vi "AI Read AFR.vi"(8 "Analog In":dbl[][](array[numeric]), 9 "Avg Point":i16[](array[numeric]), 10 "Intercept":dbl[](array[numeric]), 11 "Slope":dbl[](array[numeric])) -> (3 "Analog Out":T1)   [LabVIEW 2015]
uses:
  <vilib>/Analysis/baseanly.llb/Mean (DBL).vi
  <vilib>/Analysis/NI_AALBase.lvlib
  <vilib>/ptbypt/NI_PtbyPt.lvlib
panel:
  in  "Cluster":T1
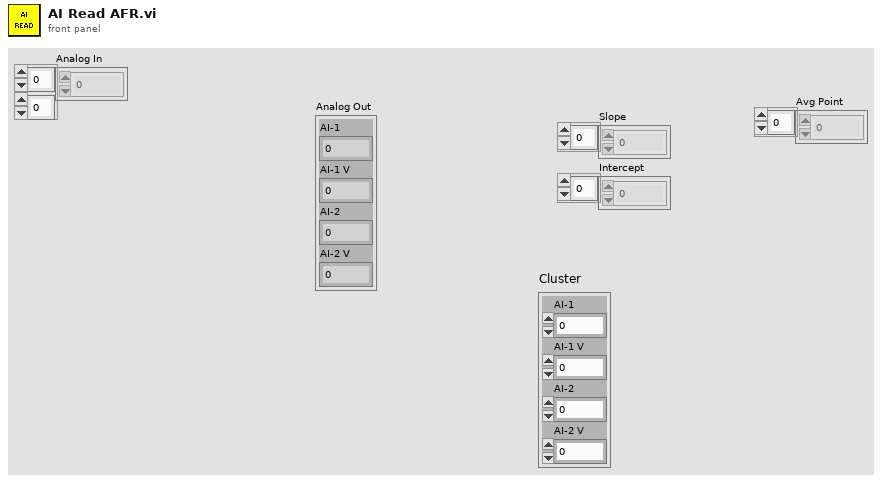
[diagram p1: front panel]
types:
  T1 = cluster{"AI-1":dbl, "AI-1 V":dbl, "AI-2":dbl, "AI-2 V":dbl}
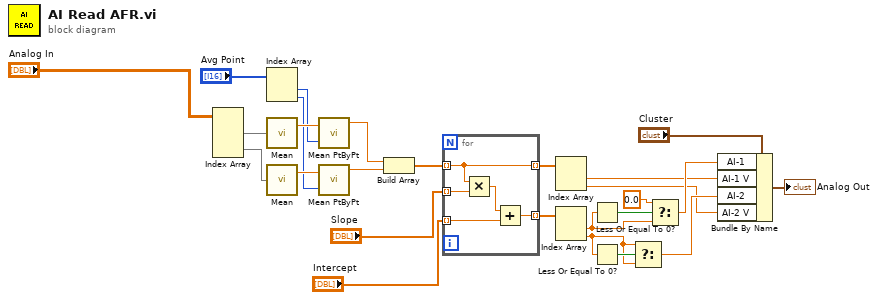
[diagram p0: block diagram]
diagram:
  n1 = Index Array(array="Analog In") -> (element #1=w4:dbl[], element #2=w3:dbl[])  [unwired: 4 in]
  n2 = Index Array(array="Avg Point") -> (element #1=w24:i16, element #2=w23:i16)  [unwired: 2 in]
  n3 = call-poly <vilib>:"Mean.vi"("X"=w4) -> ("mean"=w26:dbl)  [unwired: 1 out]
  n4 = call-poly <vilib>:"Mean.vi"("X"=w3) -> ("mean"=w25:dbl)  [unwired: 1 out]
  n5 = call <vilib>:"Mean PtByPt.vi"("x"=w26, "sample length"=w24) -> ("mean"=w18:dbl)  [unwired: 2 in, 1 out]
  n6 = call <vilib>:"Mean PtByPt.vi"("x"=w25, "sample length"=w23) -> ("mean"=w17:dbl)  [unwired: 2 in, 1 out]
  n7 = Build Array(w18, w17) -> (w19:dbl[])
  n8 = for {
    tunnel: "Slope" -> [w31] mode=indexing
    tunnel: "Intercept" -> [w29] mode=indexing
    tunnel: w19 -> [w28] mode=indexing
    tunnel: [w28] -> w14 mode=indexing
    tunnel: [w27] -> w20 mode=indexing
    n9 = Multiply(x=w28, y=w31) -> (x*y=w30:dbl)
    n10 = Add(x=w30, y=w29) -> (x+y=w27:dbl)
  }
  n11 = Index Array(array=w14) -> (element #1=w9:dbl, element #2=w8:dbl)  [unwired: 2 in]
  n12 = Index Array(array=w20) -> (element #1=w13:dbl, element #2=w5:dbl)  [unwired: 2 in]
  n13 = Less Or Equal To 0?(x=w13) -> (x <= 0?=w16:bool)
  n14 = Less Or Equal To 0?(x=w5) -> (x <= 0?=w15:bool)
  n15 = Select(t=w5, s=w15, f=w5) -> (s? t:f=w10:dbl)
  n16 = Select(t=0.0, s=w16, f=w13) -> (s? t:f=w11:dbl)
  n17 = Bundle By Name(cluster="Cluster", "AI-1"=w11, "AI-1 V"=w9, "AI-2"=w10, "AI-2 V"=w8) -> (→"Analog Out":T1)
